vi "Filter Settings by Name.vi"(8 "error in (no error)":errorcluster, 10 "name":string, 11 "settings":T1) -> (0 "error out":errorcluster, 3 "filtered settings":T1)   [LabVIEW 2017, in "DSF Core.lvlib" / "Configuration Session.lvclass"]
uses:
  Configuration Session.lvclass
  Typedefs/DSF Settings Info.ctl
  DSF Core.lvlib
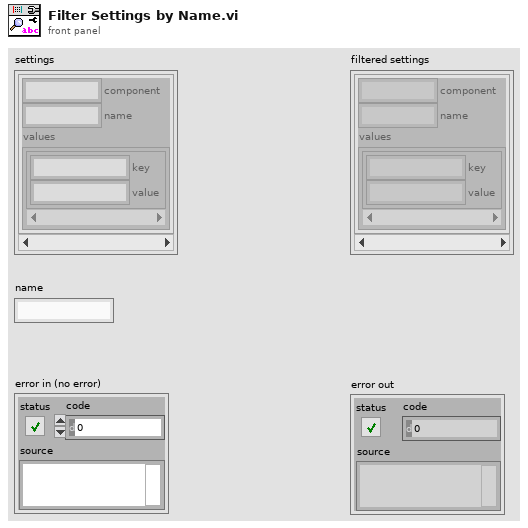
[diagram p1: front panel]
types:
  T1 = typedef "DSF Core.lvlib/DSF Settings Info.ctl" = cluster{"component":string, "name":string, "values":cluster{"key":string, "value":string}[]}[]
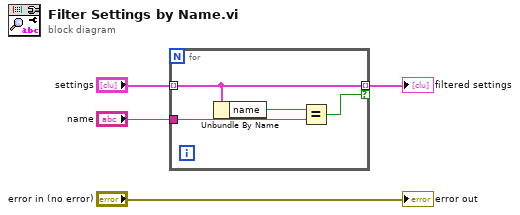
[diagram p0: block diagram]
diagram:
  n1 = for {
    tunnel: "settings" -> [w8] mode=indexing
    tunnel: [w8] -> w1 mode=indexing if=w5
    tunnel: "name" -> [w6]
    n2 = Unbundle By Name(w8) -> ("name"=w7:string)
    n3 = Equal?(x=w7, y=w6) -> (x = y?=w5:bool)
  }
  "filtered settings" <- w1
  "error out" <- "error in (no error)"
